vi "Get Parameter Value - Array of Integers.vi"(7 "Default value":i32[](array[numeric]), 8 "error in (no error)":errorcluster, 9 "Parameter name":string, 10 "Config name":string, 11 "Config in":refnum<class "Config.lvclass">) -> (0 "error out":errorcluster, 2 "Value":i32[](array[numeric]), 3 "Config out":refnum<class "Config.lvclass">)   [LabVIEW 2026, in "TALOS.lvlib" / "Classes.lvlib" / "Config.lvclass"]
doc: "Get the parameter's value (string) from the specified configuration. Use the data type terminal to specify the output type."
uses:
  Config.lvclass
  Ancestor/Ancestor/Ancestor.lvclass/Ancestor.ctl
  <vilib>/AdvancedString/Delimited String to 1D String Array (string).vi
  FGV/Error Memory/Get Error Description.vi
  Support VIs/Get PC name.vi
  Ancestor/Ancestor/Read ID.vi
  Support VIs/Get Class Name.vi
  <vilib>/Utility/error.llb/Clear Errors.vi
  FGV/Error Memory/Error Memory Core.vi
  Support VIs/Circus Root Path.vi
  FGV/Error Memory/Error Crt Lvl checker.vi
  FGV/Error Memory/Error Memory Core.vi/40c8088d-b597-4017-91af-faa98e00292e.vi
  FGV/Error Memory/Error Memory Core.vi/d4a3ab98-063c-4e44-b43d-fbdcfe6c2be2.vi
  Support VIs/Global Memory.vi
  <vilib>/Utility/LVClass/Get LV Class Name.vi
  Support VIs/Is in Packed Library.vi
  Support VIs/TALOS Root path.vi
  Support VIs/Read CSV worksheet.vi
  Support VIs/Global Constants.vi
  <vilib>/Utility/error.llb/General Error Handler.vi
  Support VIs/Error Log.vi
  Ancestor/Ancestor/Ancestor.lvclass
  <vilib>/Comparison/Equal/Equal Functor/Equal Functor.lvclass
  TALOS.lvlib
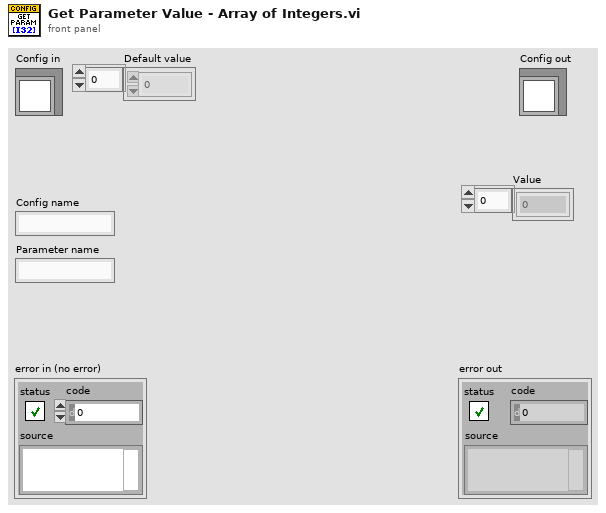
[diagram p1: front panel]
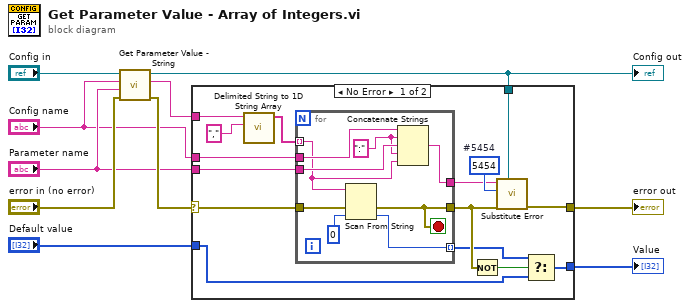
[diagram p0: block diagram]
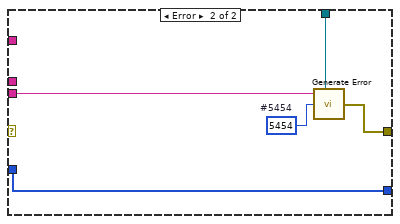
[diagram p2: hidden frame]
diagram:
  n1 = call "Get Parameter Value - String.vi"("error in (no error)"="error in (no error)", "Parameter name"="Parameter name", "Config name"="Config name", "Config in"="Config in") -> ("error out"=w8:errorcluster, "Value"=w2:string, "Config out"=w4:refnum<class "Config.lvclass">)  [unwired: 5 in]
  "Config out" <- w4
  n2 = case shown="No Error" w8 {
    selector: w8 -> [w25 _]
    tunnel: [w12 w35] -> w1
    tunnel: w4 -> [w19 w38]
    tunnel: [w18 w39] -> w7
    tunnel: "Default value" -> [w11 w35]
    tunnel: "Parameter name" -> [w24 w36]
    tunnel: "Config name" -> [w21 _]
    tunnel: w2 -> [w22 _]
    frame No Error {
      w17 = 5454  # #5454
      n3 = call-poly <vilib>:"Delimited String to 1D String Array.vi"("delimiter"=",", "delimited string"=w22) -> ("string array"=w20:string[])  [unwired: 9 in]
      n4 = for {
        tunnel: [w34] -> w13 mode=indexing
        tunnel: w24 -> [w31]
        tunnel: w21 -> [w32]
        tunnel: w20 -> [w27] mode=indexing
        tunnel: [w26] -> w15
        tunnel: [w29] -> w16
        tunnel: w25 -> [w33]
        stop <- w26 stop-if-true
        w28 = ":" ("string")
        n5 = Scan From String(input string=w27, error in=w33, default 1=0 ("default value 1")) -> (error out=w26:errorcluster, output 1=w34:i32)  [unwired: 2 in, 2 out]
        n6 = Concatenate Strings(w32, w28, w31, w28, w27) -> (w29:string)
      }
      n7 = Not(x=w15) -> (.not. x?=w14:bool)
      n8 = call "Substitute Error.vi"("LabVIEW Object"=w19, "error in (no error)"=w15, "Error Code"=w17, "Optional String"=w16) -> ("error out"=w18:errorcluster)  [unwired: 7 in]
      n9 = Select(t=w13, s=w14, f=w11) -> (s? t:f=w12:i32[])
    }
    frame Error {
      w37 = 5454  # #5454
      n10 = call "Generate Error.vi"("Optional String"=w36, "Class"=w38, "Error Code"=w37) -> ("error out"=w39:errorcluster)  [unwired: 4 in]
    }
  }
  "error out" <- w7
  "Value" <- w1
